vi "ProcessingLoop.vi"(8 "error in (no error)":errorcluster, 11 "navX - SPI_I2C ProcessingLoop in":refnum<class "navX - SPI_I2C ProcessingLoop.lvclass">) -> (0 "error out":errorcluster, 3 "navX - SPI_I2C ProcessingLoop out":refnum<class "navX - SPI_I2C ProcessingLoop.lvclass">)   [LabVIEW 2015, in "navX Library v3.lvlib" / "navX - SPI_I2C ProcessingLoop.lvclass"]
uses:
  navX - SPI_I2C ProcessingLoop.lvclass
  navX Error Status/navX Error Status.lvclass
  navX - Interface/navX - Interface.lvclass/navX - Interface.ctl
  <vilib>/Platform/TimedLoop/XDataNode/timing_clust.ctl
  <vilib>/Platform/TimedLoop/XDataNode/nitl_modes.ctl
  <vilib>/Platform/TimedLoop/XDataNode/wakeup.ctl
  navX - Interface/navX - Interface.lvclass
  <vilib>/platform/TimedLoop/XDataNode/XDataNode.xnode
  <vilib>/Platform/TimedLoop/XDataNode/XDNodeRunTimeDep.lvlib
panel:
  out "Iteration Duration":i64
  out "Finished Late? [i-1]":bool
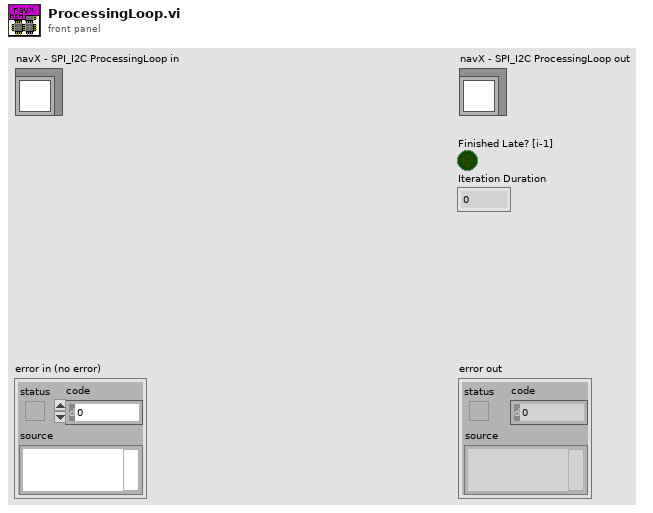
[diagram p1: front panel]
types:
  T1 = typedef "XDNodeRunTimeDep.lvlib/timing_clust.ctl" = cluster{"Expected End [f-1]":u64, "Actual End [f-1]":u64, "Finished Late? [f-1]":bool, "Expected End [i-1]":u64, "Actual End [i-1]":u64, "Finished Late? [i-1]":bool, "Expected Start [i]":u64, "Actual Start [i]":u64, "Expected Start [f]":u64, "Actual Start [f]":u64, "Source Name":string, "Structure Name":string, "Period":i64, "Deadline":i64, "Offset":i64, "Start":i64, "Priority":i32, "Timeout":i32, "Mode":T2, "Wakeup Reason":T3, "Error":errorcluster, "Source Type":string, "Secondary Source Type":string, "Global End Time":u64, "Global Start Time":u64, "Frame Duration":u64, "Iteration Duration":u64, "Assigned CPU":i32, "I/O Scan Engine Mode":u32}
  T2 = typedef "XDNodeRunTimeDep.lvlib/nitl_modes.ctl" = enum32{"No Change", "Process missed periods, maintain original phase", "Discard missed periods, maintain original phase", "Process missed periods, ignore original phase", "Discard missed periods, ignore original phase"}
  T3 = typedef "XDNodeRunTimeDep.lvlib/wakeup.ctl" = enum32{"Normal", "Aborted", "Asynchronous wakeup", "Timing source error", "Timed loop error", "Timeout"}
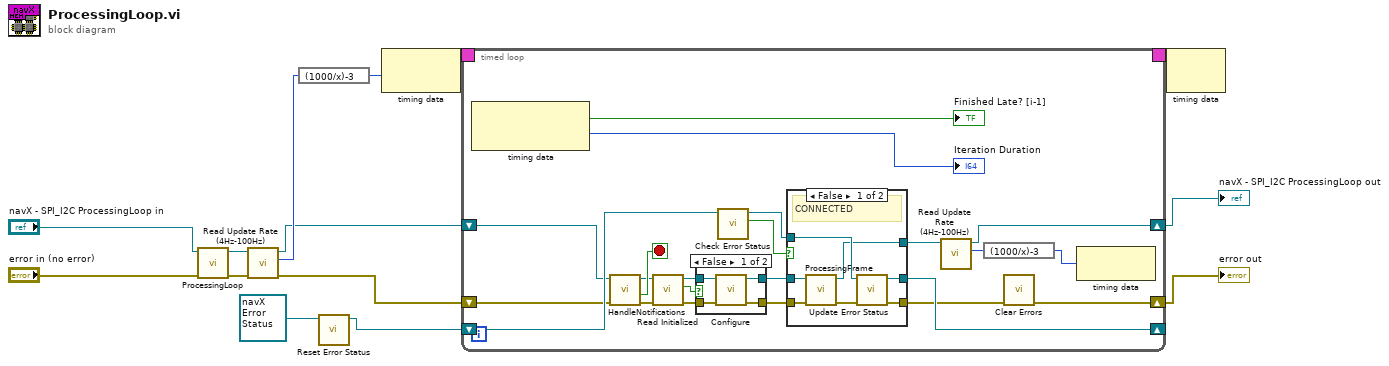
[diagram p0: block diagram]
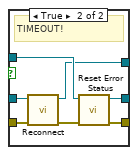
[diagram p3: hidden frame]
diagram:
  n1 = call-parent "ProcessingLoop.vi"("error in (no error)"="error in (no error)", "navX - Interface in"="navX - SPI_I2C ProcessingLoop in") -> ("error out"=w1:errorcluster, "navX - Interface out"=w3:refnum<class "navX - SPI_I2C ProcessingLoop.lvclass">)  [unwired: 8 in]
  n2 = call "Read Update Rate (4Hz-100Hz).vi"("error in (no error)"=w1, "navX - Interface in"=w3) -> ("error out"=w5:errorcluster, "Update Rate (4Hz-100Hz)"=w8:u8, "navX - Interface out"=w7:refnum<class "navX - SPI_I2C ProcessingLoop.lvclass">)  [unwired: 7 in]
  n3 = expression code="(1000/x)-3"(w8) -> (w6:u8)
  n4 = call "Reset Error Status.vi"("navX Error Status in"=refnum<class "navX Error Status.lvclass"> refnum ("navX Library v3.lvlib:navX Error Status.lvclass")) -> ("navX Error Status out"=w11:refnum<class "navX Error Status.lvclass">)  [unwired: 9 in, 1 out]
  n5 = node-c288(w6) -> (w14:T1)
  n6 = timed-loop {
    timing: w14 -> [_]
    timing-out: [_] -> w13
    shift-right: [w25] -> w10
    shift-left: w7 -> [w24]
    shift-right: [w29] -> w9
    shift-left: w5 -> [w27]
    shift-right: [w32] -> _
    shift-left: w11 -> [w35]
    stop <- w28 stop-if-true
    n7 = node-c288() -> (→"Finished Late? [i-1]":bool, →"Iteration Duration":i64)  [unwired: 1 in]
    n8 = call "HandleNotifications.vi"("error in (no error)"=w27, "navX - Interface in"=w24) -> ("error out"=w26:errorcluster, "Halt?"=w28:bool, "navX - Interface out"=w23:refnum<class "navX - SPI_I2C ProcessingLoop.lvclass">)  [unwired: 7 in]
    n9 = call "Read Initialized.vi"("error in (no error)"=w26, "navX - Interface in"=w23) -> ("error out"=w20:errorcluster, "Initialized?"=w19:bool, "navX - Interface out"=w21:refnum<class "navX - SPI_I2C ProcessingLoop.lvclass">)  [unwired: 7 in]
    n10 = case shown="False" w19 {
      tunnel: [w40 w41] -> w18
      tunnel: [w39 w42] -> w17
      tunnel: w21 -> [w38 w42]
      tunnel: w20 -> [w37 w41]
      frame False {
        n11 = call-dynamic "Configure.vi"("error in (no error)"=w37, "navX - Interface in"=w38) -> ("error out"=w40:errorcluster, "navX - Interface out"=w39:refnum<class "navX - SPI_I2C ProcessingLoop.lvclass">)  [unwired: 8 in]
      }
      frame True {
      }
    }
    n12 = call "Check Error Status.vi"("navX Error Status in"=w35) -> ("Timeout!"=w34:bool, "navX Error Status out"=w33:refnum<class "navX Error Status.lvclass">)  [unwired: 8 in, 1 out]
    n13 = case shown="False" w34 {
      tunnel: w33 -> [w46 w56]
      tunnel: w17 -> [w49 w51]
      tunnel: w18 -> [w48 w54]
      tunnel: [w45 w55] -> w32
      tunnel: [w44 w52] -> w30
      tunnel: [w43 w50] -> w31
      frame False {
        # "CONNECTED"
        n14 = call-dynamic "ProcessingFrame.vi"("error in (no error)"=w48, "navX - Interface in"=w49) -> ("error out"=w47:errorcluster, "navX - Interface out"=w43:refnum<class "navX - SPI_I2C ProcessingLoop.lvclass">)  [unwired: 8 in]
        n15 = call "Update Error Status.vi"("error in (no error)"=w47, "navX Status in"=w46) -> ("error out"=w44:errorcluster, "navX Status out"=w45:refnum<class "navX Error Status.lvclass">)  [unwired: 7 in, 1 out]
      }
      frame True {
        # "TIMEOUT!"
        n16 = call-dynamic "Reconnect.vi"("error in (no error)"=w54, "navX - Interface in"=w51) -> ("error out"=w53:errorcluster, "navX - Interface out"=w50:refnum<class "navX - SPI_I2C ProcessingLoop.lvclass">)  [unwired: 8 in]
        n17 = call "Reset Error Status.vi"("error in (no error)"=w53, "navX Error Status in"=w56) -> ("error out"=w52:errorcluster, "navX Error Status out"=w55:refnum<class "navX Error Status.lvclass">)  [unwired: 8 in]
      }
    }
    n18 = call "Read Update Rate (4Hz-100Hz).vi"("navX - Interface in"=w31) -> ("Update Rate (4Hz-100Hz)"=w36:u8, "navX - Interface out"=w25:refnum<class "navX - SPI_I2C ProcessingLoop.lvclass">)  [unwired: 8 in, 1 out]
    n19 = expression code="(1000/x)-3"(w36) -> (w22:u8)
    n20 = call <vilib>:"Clear Errors.vi"("error in (no error)"=w30) -> ("error out"=w29:errorcluster)  [unwired: 5 in, 1 out]
    n21 = node-c288(w22) -> ()  [unwired: 1 out]
  }
  "error out" <- w9
  "navX - SPI_I2C ProcessingLoop out" <- w10
  n22 = node-c288(w13) -> ()  [unwired: 1 out]
